vi "devidePhases.vi"(0 "reference in":refnum<class "subject.lvclass">, 5 "error in (no error)":errorcluster) -> (14 "reference out":refnum<class "subject.lvclass">, 19 "error out":errorcluster)   [LabVIEW 2015, in "subject.lvclass"]
uses:
  subject.lvclass
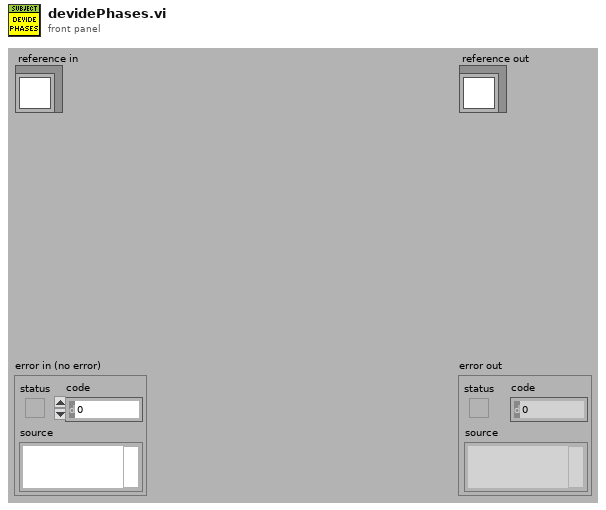
[diagram p1: front panel]
types:
  T1 = typedef "subject.lvclass/ObjectAttributesRef.ctl" = refnum<data-value>
  T2 = typedef "subject.lvclass/ObjectAttributes.ctl" = cluster{"MyAttribute":dbl, "data":cluster{"Ve_warm":dbl[], "time_warm":dbl[], "name":string, "phase":dbl[], "VCO2":dbl[], "VO2":dbl[], "PetCO2":dbl[], "RQ":dbl[], "HR":dbl[], "Ve_warm_inter":dbl[], "time_warm_inter":dbl[], "Ve_exer":dbl[], "time_exer":dbl[], "Ve_exer_inter":dbl[], "time_exer_inter":dbl[], "Ve":dbl[], "time":dbl[], "Ve_exer_inter_filtered":dbl[], "Ve_warm_inter_filtered":dbl[]}, "results_5l":cluster{"EOV":bool, "osci_amplitude":dbl[], "osci_width":dbl[], "peak_location":dbl[], "threshold":dbl, "width":i32}, "results_15percent":cluster{"EOV":bool, "osci_amplitude":dbl[], "osci_width":dbl[], "peak_location":dbl[], "threshold":dbl, "width":i32}, "supportData":cluster{"peaksAmplitude":dbl[], "iPeaksLocation":dbl[], "valesAmplitude":dbl[], "iValesLocation":dbl[], "threshold":dbl, "meanAmpl_warm":i32, "#_peaks":i32, "width":i32}, "results_user_selection":cluster{"EOV":bool, "osci_amplitude":dbl[], "osci_width":dbl[], "peak_location":dbl[], "threshold":dbl, "width":i32}, "results_warm_up":cluster{"EOV":bool, "osci_amplitude":dbl[], "osci_width":dbl[], "peak_location":dbl[], "threshold":dbl, "width":i32}}
  T3 = cluster{"Ve_warm":dbl[], "time_warm":dbl[], "name":string, "phase":dbl[], "VCO2":dbl[], "VO2":dbl[], "PetCO2":dbl[], "RQ":dbl[], "HR":dbl[], "Ve_warm_inter":dbl[], "time_warm_inter":dbl[], "Ve_exer":dbl[], "time_exer":dbl[], "Ve_exer_inter":dbl[], "time_exer_inter":dbl[], "Ve":dbl[], "time":dbl[], "Ve_exer_inter_filtered":dbl[], "Ve_warm_inter_filtered":dbl[]}
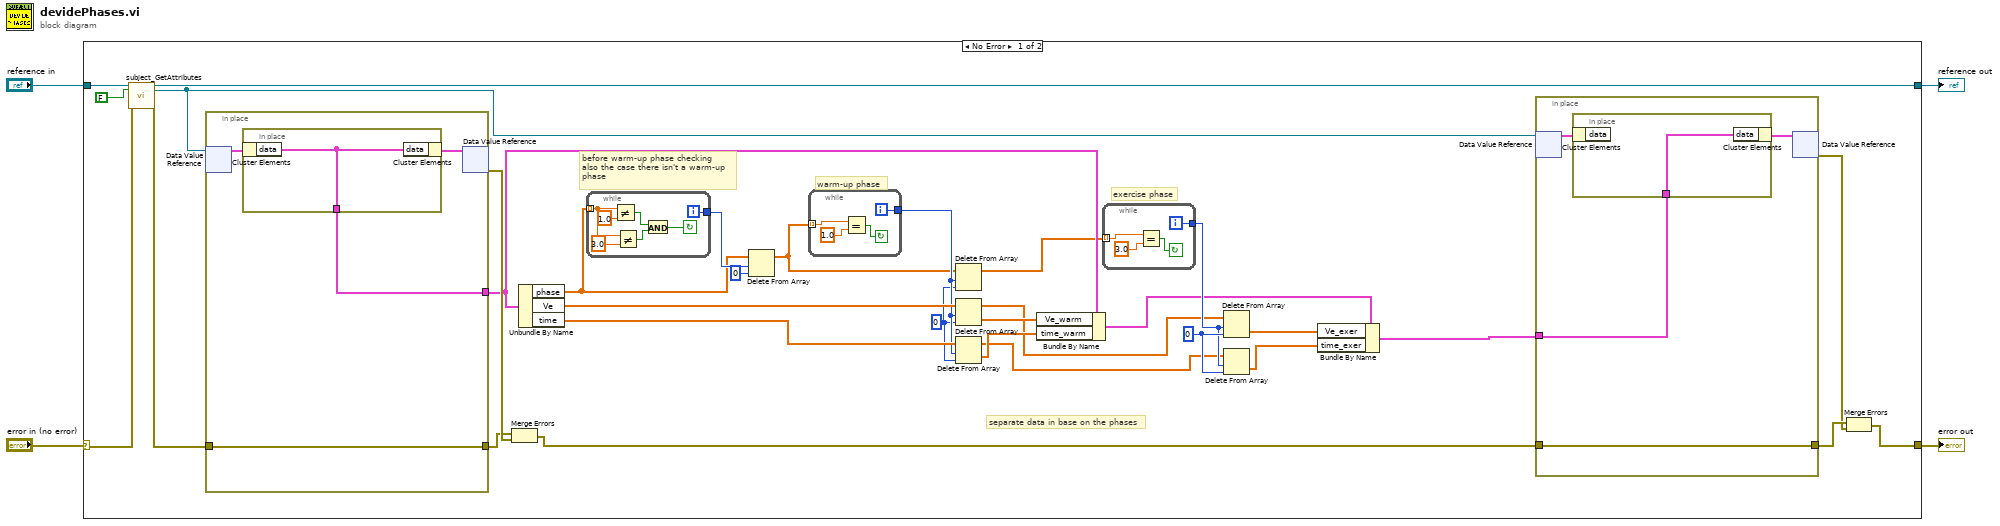
[diagram p0: block diagram]
diagram:
  n1 = case shown="No Error" "error in (no error)" {
    selector: "error in (no error)" -> [w32 w63]
    tunnel: [w16 w63] -> w3
    tunnel: [w30 w62] -> w1
    tunnel: "reference in" -> [w34 w62]
    frame No Error {
      w24 = 0 ("index")
      w26 = 0 ("index")
      # "before warm-up phase checking\nalso the case there isn't a warm-up\nphase"
      # "separate data in base on the phases"
      # "exercise phase"
      # "warm-up phase"
      n2 = call "subject_GetAttributes.vi"("reference in"=w34, "return data? (T)"=FALSE, "error in (no error)"=w32) -> ("reference out"=w30:refnum<class "subject.lvclass">, "attributes ref"=w20:T1, "error out"=w31:errorcluster)  [unwired: 13 in, 1 out]
      n3 = in-place {
        in-place-border: w31 -> [w58]
        in-place-border: [w58] -> w35
        in-place-border: [w57] -> w25
        n4 = in-place-dvr #1(w20) -> (w59:T2)  [unwired: 1 out]
        n5 = in-place {
          in-place-border: [w61] -> w57
          n6 = in-place-cluster #2(w59) -> ("data"=w61:T3)
          n7 = in-place-cluster #2("data"=w61) -> (w60:T2)
        }
        n8 = in-place-dvr #1(w60) -> (w36:errorcluster)  [unwired: 1 out]
      }
      n9 = Merge Errors(w35, w36) -> (w21:errorcluster)
      n10 = Unbundle By Name(w25) -> ("phase"=w6:dbl[], "Ve"=w29:dbl[], "time"=w28:dbl[])
      n11 = while {
        tunnel: w6 -> [w41] mode=indexing
        tunnel: [w43] -> w8
        i -> [w43]
        stop <- w37 continue-if-true
        n12 = Not Equal?(x=w41, y=1.0) -> (x != y?=w38:bool)
        n13 = Not Equal?(x=w41, y=3.0) -> (x != y?=w39:bool)
        n14 = And(x=w38, y=w39) -> (x .and. y?=w37:bool)
      }
      n15 = Delete From Array(array=w6, length=w8, index=0) -> (array with subset deleted=w5:dbl[])  [unwired: 1 out]
      n16 = while {
        tunnel: w5 -> [w56] mode=indexing
        tunnel: [w55] -> w27
        i -> [w55]
        stop <- w54 continue-if-true
        n17 = Equal?(x=w56, y=1.0) -> (x = y?=w54:bool)
      }
      n18 = Delete From Array(array=w5, length=w27, index=w26) -> (array with subset deleted=w15:dbl[])  [unwired: 1 out]
      n19 = Delete From Array(array=w29, length=w27, index=w26) -> (deleted portion=w14:dbl[], array with subset deleted=w12:dbl[])
      n20 = Delete From Array(array=w28, length=w27, index=w26) -> (deleted portion=w13:dbl[], array with subset deleted=w11:dbl[])
      n21 = Bundle By Name(cluster=w25, "Ve_warm"=w14, "time_warm"=w13) -> (w22:T3)
      n22 = while {
        tunnel: w15 -> [w52] mode=indexing
        tunnel: [w51] -> w23
        i -> [w51]
        stop <- w50 continue-if-true
        n23 = Equal?(x=w52, y=3.0) -> (x = y?=w50:bool)
      }
      n24 = Delete From Array(array=w12, length=w23, index=w24) -> (deleted portion=w10:dbl[])  [unwired: 1 out]
      n25 = Delete From Array(array=w11, length=w23, index=w24) -> (deleted portion=w9:dbl[])  [unwired: 1 out]
      n26 = Bundle By Name(cluster=w22, "Ve_exer"=w10, "time_exer"=w9) -> (w19:T3)
      n27 = in-place {
        in-place-border: w21 -> [w45]
        in-place-border: [w45] -> w18
        in-place-border: w19 -> [w44]
        n28 = in-place-dvr #3(w20) -> (w46:T2)  [unwired: 1 out]
        n29 = in-place {
          in-place-border: w44 -> [w48]
          n30 = in-place-cluster #4(w46) -> ()  [unwired: 1 out]
          n31 = in-place-cluster #4("data"=w48) -> (w47:T2)
        }
        n32 = in-place-dvr #3(w47) -> (w17:errorcluster)  [unwired: 1 out]
      }
      n33 = Merge Errors(w18, w17) -> (w16:errorcluster)
    }
    frame Error {
    }
  }
  "error out" <- w3
  "reference out" <- w1
